vi "Build All Versions.vi"() -> ()   [LabVIEW 2020]
doc: "This VI will automatically build all TWM version (different driver sets)."
uses:
  Build Setup.ctl
  1a084e9b-14bd-426b-b511-56d3df6ad0ad.vi
  <vilib>/Utility/error.llb/Error Cluster From Error Code.vi
  <vilib>/AppBuilder/AB_API_Simple/Get Build Specification Version (path).vi
  <vilib>/AppBuilder/AB_API_Simple/Set Build Specification Version (path).vi
  <vilib>/Comparison/Equal/Equal Functor/Equal Functor.lvclass
  <vilib>/ErrorRing/Error Ring.xnode
  <vilib>/AppBuilder/AB_API_Simple/NI_App_Builder_API.lvlib
panel:
  out "Status":string
  in  "btn all":bool
  in  "builds":i32[](listbox) caption="Available build variants (different driver sets):"
  in  "Target Name":string="My Computer"
  in  "Build Specification Name (the full equiped version)":string="Open-Z-bridge-full"
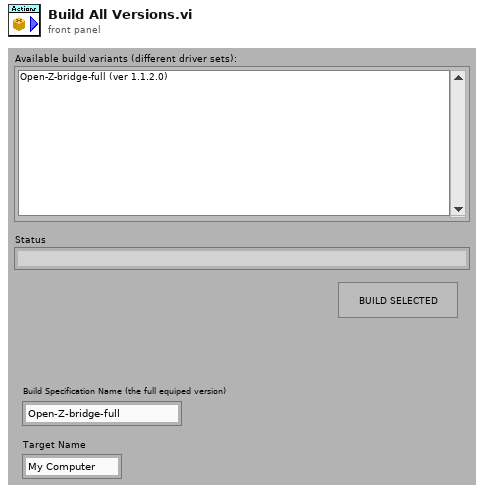
[diagram p1: front panel]
types:
  T1 = typedef "Build Setup.ctl" = cluster{"project path":path, "build spec name":string, "target name":string}
  T2 = typedef "NI_App_Builder_API.lvlib/Build Specification Version.ctl" = cluster{"Major":u16, "Minor":u16, "Fix":u16, "Build":u16}
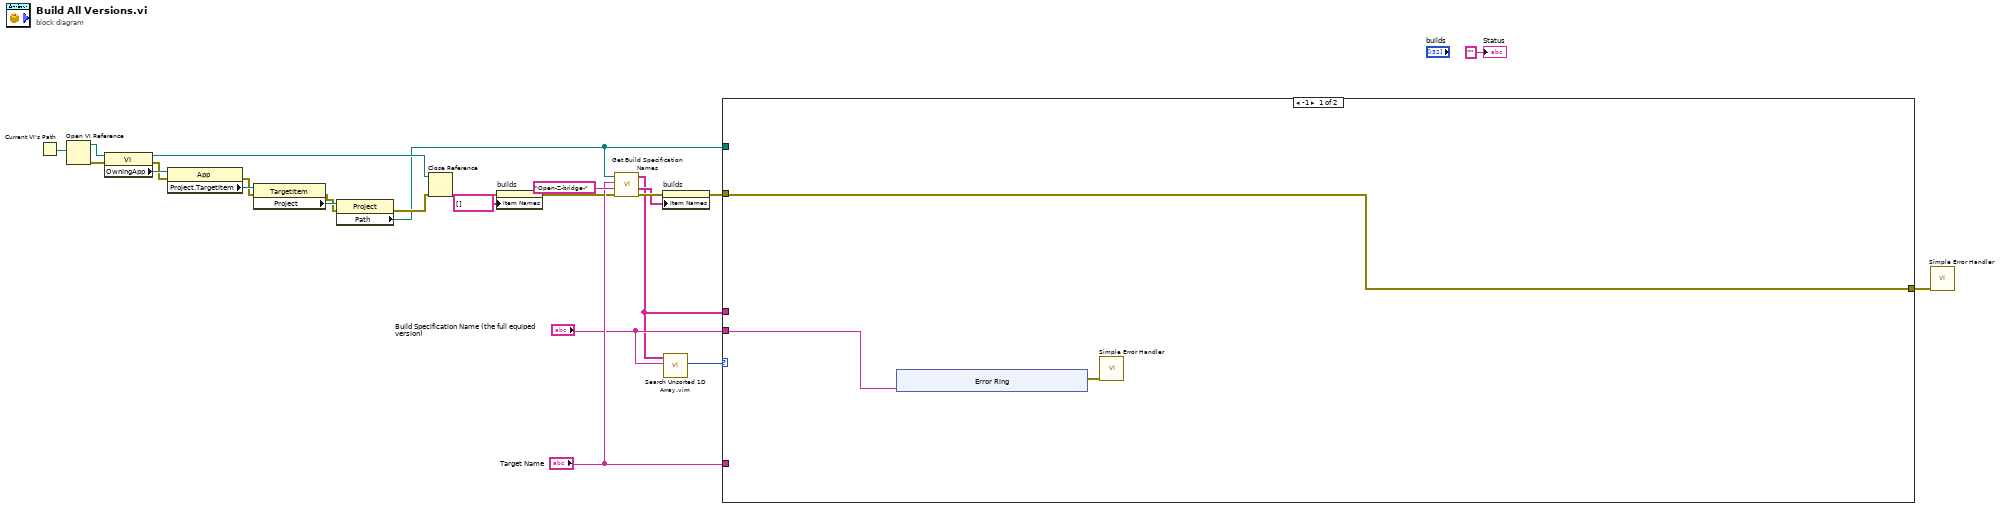
[diagram p0: block diagram]
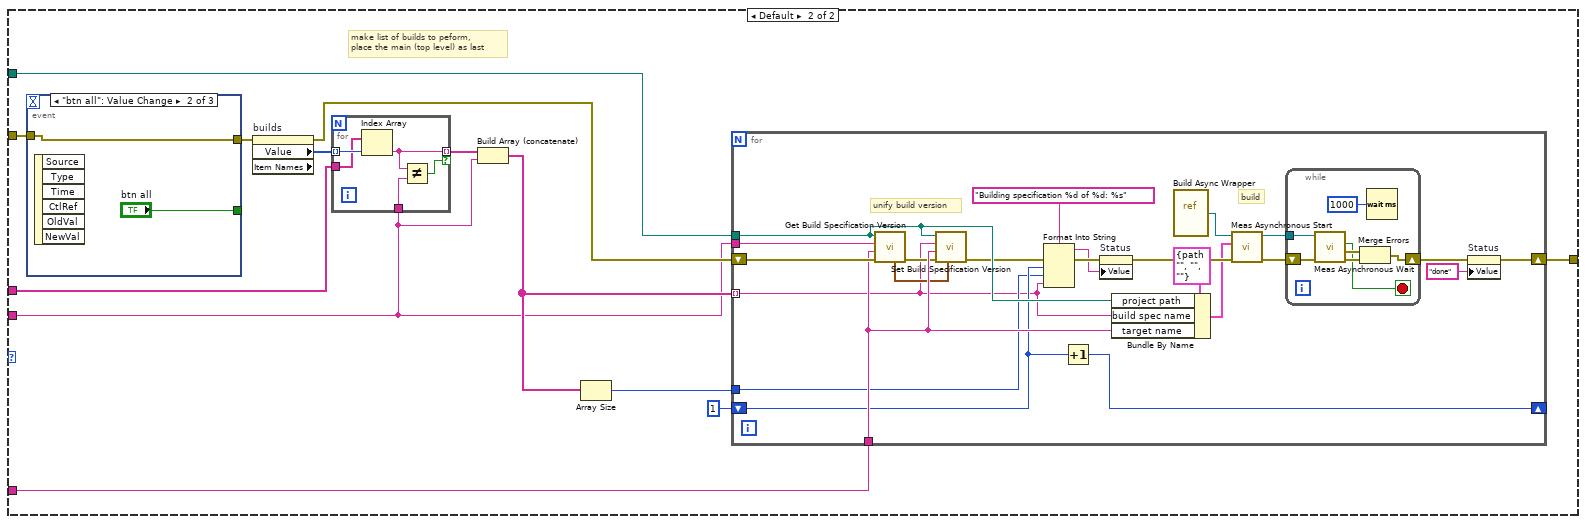
[diagram p2: hidden frame]
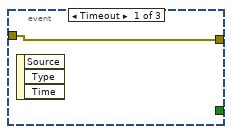
[diagram p3: hidden frame]
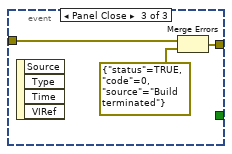
[diagram p4: hidden frame]
diagram:
  n1 = Current VI's Path() -> (path=w19:path)
  n2 = Open VI Reference(vi path=w19) -> (vi reference=w17:refnum<vi>, error out=w18:errorcluster)  [unwired: 5 in]
  n3 = property class="VI"(reference=w17, error in=w18) -> (reference out=w12:refnum<vi>, error out=w15:errorcluster, "OwningApp"=w16:refnum<vi>)
  n4 = property class="App"(reference=w16, error in=w15) -> (error out=w13:errorcluster, "Project.TargetItem"=w14:refnum<vi>)  [unwired: 1 out]
  n5 = property class="TargetItem"(reference=w14, error in=w13) -> (error out=w8:errorcluster, "Project"=w9:refnum<vi>)  [unwired: 1 out]
  n6 = property class="Project"(reference=w9, error in=w8) -> (error out=w7:errorcluster, "Path"=w6:path)  [unwired: 1 out]
  n7 = Close Reference(reference=w12, error in (no error)=w7) -> (error out=w3:errorcluster)
  n8 = property on="builds" class="LstBox (strict)"(error in=w3, "Item Names"=string[] []) -> (error out=w2:errorcluster)  [unwired: 1 in, 1 out]
  n9 = call "Get Build Specification Names.vi"("error in (no error)"=w2, "Build specification regexp filter (.*)"="Open-Z-bridge-", "Target Name"="Target Name", "Project Path"=w6) -> ("error out"=w24:errorcluster, "Build specification names with version string"=w21:string[], "Build specification names"=w5:string[])  [unwired: 3 in, 2 out]
  n10 = property on="builds" class="LstBox (strict)"(error in=w24, "Item Names"=w21) -> (error out=w23:errorcluster)  [unwired: 1 in, 1 out]
  n11 = call "Search Unsorted 1D Array.vim"("element"="Build Specification Name (the full equiped version)", "unsorted 1D array"=w5) -> ("index of element"=w10:i32)  [unwired: 9 in]
  n12 = case shown="-1" w10 {
    tunnel: [w28 w36] -> w4
    tunnel: w23 -> [w28 w48]
    tunnel: "Target Name" -> [_ w41]
    tunnel: w6 -> [_ w40]
    tunnel: "Build Specification Name (the full equiped version)" -> [w26 w38]
    tunnel: w5 -> [_ w37]
    frame -1 {
      n13 = xnode "Error Ring"("parameter 0"=w26) -> ("error out"=w27:errorcluster)
      n14 = call <vilib>:"Simple Error Handler.vi"("error in (no error)"=w27) -> ()  [unwired: 4 in, 5 out]
    }
    frame Default {
      # "make list of builds to peform,\nplace the main (top level) as last"
      n15 = event shown="[1] \"btn all\": Value Change" {
        selector: _ -> [_ _ _]
        dyn-events: _ -> [_ _ _]
        timeout: _ -> [_ _ _]
        tunnel: w48 -> [w84 w85 w89]
        tunnel: [w84 w85 w87] -> w47
        tunnel: [_ "btn all" _] -> _
        event Timeout {
          n16 = event-data() -> ()  [unwired: 1 in, 3 out]
        }
        event "btn all": Value Change {
          n17 = event-data() -> ()  [unwired: 1 in, 6 out]
        }
        event Panel Close {
          n18 = event-data() -> ()  [unwired: 1 in, 4 out]
          n19 = Merge Errors(w89, errorcluster {"status"=TRUE, "code"=0, "source"="Build terminated"} ("error in")) -> (w87:errorcluster)
        }
      }
      n20 = property on="builds" class="LstBox (strict)" props=["Value", "Item Names"](error in=w47) -> (error out=w45:errorcluster, "Value"=w46:i32[])  [unwired: 1 in, 2 out]
      n21 = for {
        tunnel: w46 -> [w83] mode=indexing
        tunnel: w37 -> [w82]
        tunnel: w38 -> [w81]
        tunnel: [w80] -> w43 mode=indexing if=w79
        n22 = Index Array(array=w82, index=w83) -> (element=w80:string)
        n23 = Not Equal?(x=w80, y=w81) -> (x != y?=w79:bool)
      }
      n24 = Build Array (concatenate)(w43, w38) -> (w42:string[])
      n25 = Array Size(array=w42) -> (size(s)=w44:i32)
      n26 = for {
        tunnel: w40 -> [w70]
        tunnel: w38 -> [w69]
        tunnel: w41 -> [w68]
        tunnel: w42 -> [w49] mode=indexing
        tunnel: w44 -> [w50]
        shift-right: [w67] -> _
        shift-left: 1 -> [w51]
        shift-right: [w66] -> w36
        shift-left: w45 -> [w71]
        # "build"
        # "unify build version"
        n27 = call-poly <vilib>:"Get Build Specification Version.vi"("error in (no error)"=w71, "Name of target (My Computer)"=w68, "Name of build specification"=w69, "Path to project"=w70) -> ("error out"=w65:errorcluster, "Build Specification Version"=w64:T2)  [unwired: 6 in]
        n28 = call-poly <vilib>:"Set Build Specification Version.vi"("Build Specification Version"=w64, "error in (no error)"=w65, "Name of target (My Computer)"=w68, "Name of build specification"=w49, "Path to project"=w70) -> ("error out"=w62:errorcluster)  [unwired: 6 in]
        n29 = Format Into String(format string="Building specification %d of %d: %s", error in=w62, w51, w50, w49) -> (resulting string=w60:string, error out=w63:errorcluster)  [unwired: 1 in]
        n30 = Increment(x=w51) -> (x+1=w67:i32)
        n31 = property on="Status" class="Str"(error in=w63, "Value"=w60) -> (error out=w58:errorcluster)  [unwired: 1 in, 1 out]
        n32 = Bundle By Name(cluster=T1 {"project path"=path "", "build spec name"="", "target name"=""} ("build setup"), "project path"=w70, "build spec name"=w49, "target name"=w68) -> (w56:T1)
        n33 = vi-ref "Build Async Wrapper.vi"() -> (w55:refnum<vi>)
        n34 = call "Meas Asynchronous Start.vi"("error in"=w58, "parameter in"=w56, "Static VI reference in (empty)"=w55) -> ("error out"=w54:errorcluster, "async VI reference out"=w53:refnum<vi>)  [unwired: 7 in]
        n35 = while {
          tunnel: w53 -> [w77]
          shift-right: [w74] -> w52
          shift-left: w54 -> [w78]
          stop <- w73 stop-if-true
          n36 = call "Meas Asynchronous Wait.vi"("error in"=w78, "VI reference (empty)"=w77) -> ("error out"=w76:errorcluster, "VI's error out"=w75:errorcluster, "VI returned?"=w73:bool)  [unwired: 5 in, 2 out]
          n37 = Merge Errors(w75, w76) -> (w74:errorcluster)
          n38 = Wait (ms)(milliseconds to wait=u32 1000) -> ()  [unwired: 1 out]
        }
        n39 = property on="Status" class="Str"(error in=w52, "Value"="done" ("Status")) -> (error out=w66:errorcluster)  [unwired: 1 in, 1 out]
      }
    }
  }
  n40 = call <vilib>:"Simple Error Handler.vi"("error in (no error)"=w4) -> ()  [unwired: 4 in, 5 out]
  "Status" <- "" ("Status")
